vi "test.vi"() -> ()   [LabVIEW 2020]
panel:
  out "Batch Length":i32
  out "Actual Bitrate kHz 2":i32=1000
  in  "SDI":u64[](array[numeric]) format="%.0x"
  out "dup Cheetah Handle":i32
  out "Total Shifted Out":i32
  out "Actual Bitrate kHz":i32=1000
  out "error out":errorcluster
  in  "Rds per Sec":dbl=2000.0 max=2000000000.0
  out "SDO":u64[](array[numeric]) format="%x"
  in  "SCLK (kHz)":i32=2000 min=0
  out "Cheetah Handle":i32
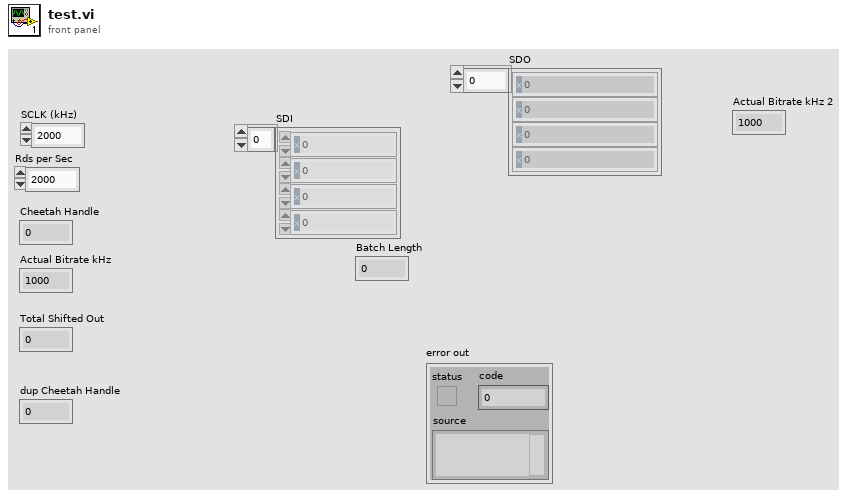
[diagram p1: front panel]
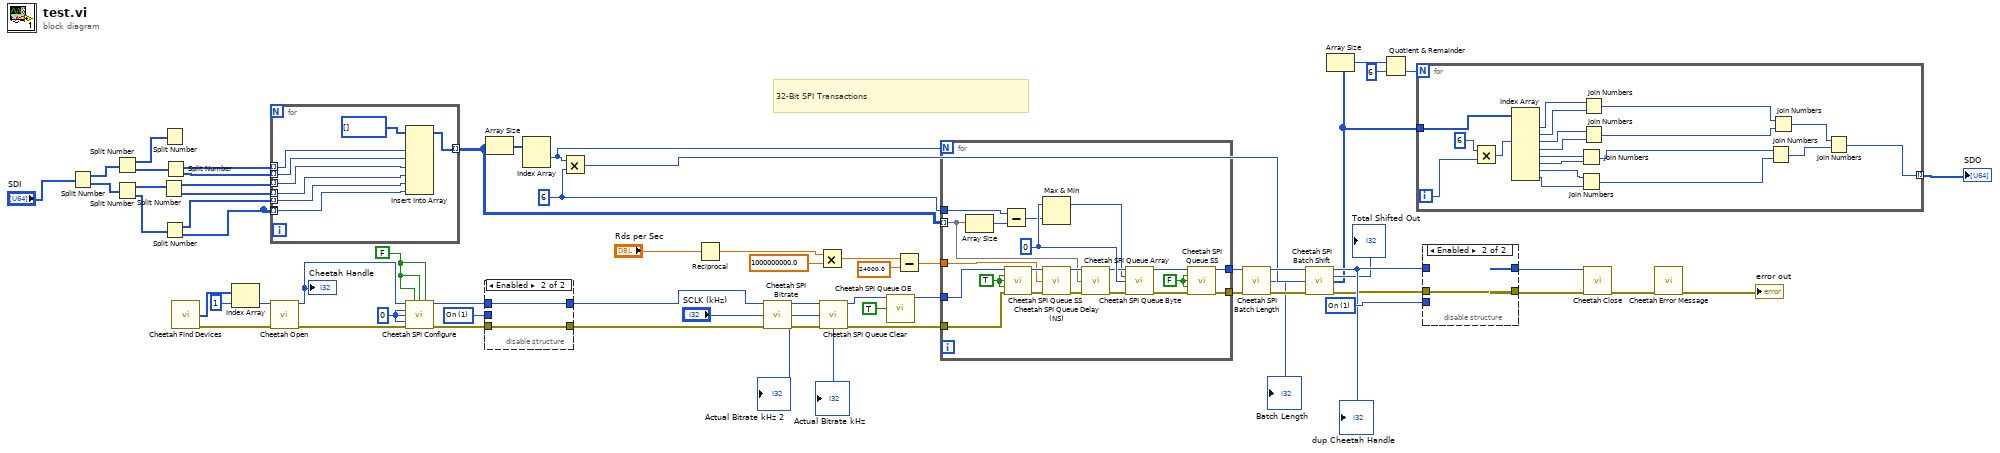
[diagram p0: block diagram]
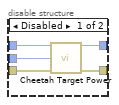
[diagram p2: hidden frame]
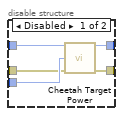
[diagram p3: hidden frame]
diagram:
  w18 = 6 ("y")
  w43 = u16 1 items=["Off", "On", "Query"] ("Requested Configuration (2: Query)")
  w44 = u16 1 items=["Off", "On", "Query"] ("Requested Configuration (2: Query)")
  w59 = FALSE
  w61 = 0
  # "32-Bit SPI Transactions"
  n1 = Split Number(x="SDI") -> (hi(x)=w29:u32[], lo(x)=w28:u32[])
  n2 = Split Number(x=w29) -> (hi(x)=w5:u16[], lo(x)=w4:u16[])
  n3 = Split Number(x=w28) -> (hi(x)=w8:u16[], lo(x)=w7:u16[])
  n4 = Split Number(x=w8) -> (hi(x)=w12:u8[], lo(x)=w11:u8[])
  n5 = Split Number(x=w5) -> ()  [unwired: 2 out]
  n6 = Split Number(x=w7) -> (hi(x)=w10:u8[], lo(x)=w9:u8[])
  n7 = Split Number(x=w4) -> (hi(x)=w3:u8[], lo(x)=w2:u8[])
  n8 = call <instrlib>:"Cheetah Find Devices.vi"() -> ("Ports"=w62:u16[], "error out"=w58:errorcluster)  [unwired: 13 in, 1 out]
  n9 = Index Array(array=w62, index=1) -> (element=w50:u16)
  n10 = for {
    tunnel: w12 -> [w67] mode=indexing
    tunnel: [w71] -> w27 mode=indexing
    tunnel: w10 -> [w65] mode=indexing
    tunnel: w9 -> [w64] mode=indexing
    tunnel: w9 -> [_] mode=indexing
    tunnel: w11 -> [w66] mode=indexing
    tunnel: w3 -> [w69] mode=indexing
    tunnel: w2 -> [w68] mode=indexing
    n11 = Insert Into Array(array=u8[] [], new element #1=w69, new element #2=w68, new element #3=w67, new element #4=w66, new element #5=w65, new element #6=w64) -> (w71:u8[])  [unwired: 1 in]
  }
  n12 = call <instrlib>:"Cheetah Open.vi"("Port Number (0)"=w50, "error in (no error)"=w58) -> ("Cheetah Handle"=w55:i32, "error out"=w57:errorcluster)  [unwired: 12 in]
  "Cheetah Handle" <- w55
  n13 = call <instrlib>:"Cheetah SPI Configure.vi"("Cheetah Handle"=w55, "SS0 Active High? (False)"=w59, "SS1 Active High? (False)"=w59, "SS2 Active High? (False)"=w59, "Polarity (0: Rising/Falling)"=w61, "Phase (0: Sample/Setup)"=w61, "Bitorder (0: MSB)"=w61, "error in (no error)"=w57) -> ("dup Cheetah Handle"=w54:i32, "error out"=w56:errorcluster)  [unwired: 6 in]
  n14 = disable-structure shown="Enabled" {
    disable-tunnel: w56 -> [w76 w77]
    disable-tunnel: w54 -> [w75 w78]
    disable-tunnel: [w74 w77] -> w53
    disable-tunnel: [w73 w78] -> w51
    disable-tunnel: w43 -> [w72 _]
    frame Disabled {
      n15 = call <instrlib>:"Cheetah Target Power.vi"("Cheetah Handle"=w75, "Requested Configuration (2: Query)"=w72, "error in (no error)"=w76) -> ("dup Cheetah Handle"=w73:i32, "error out"=w74:errorcluster)  [unwired: 10 in, 1 out]
    }
    frame Enabled {
    }
  }
  n16 = Array Size(array=w27) -> (size(s)=w42:i32[])
  n17 = Index Array(array=w42) -> (element #1=w14:i32)  [unwired: 2 in, 1 out]
  n18 = Multiply(x=w14, y=w18) -> (x*y=w13:i32)
  n19 = Reciprocal(x="Rds per Sec") -> (1/x=w20:dbl)
  n20 = call <instrlib>:"Cheetah SPI Bitrate.vi"("Cheetah Handle"=w51, "Requested Bitrate kHz (1000)"="SCLK (kHz)", "error in (no error)"=w53) -> ("dup Cheetah Handle"=w49:i32, "Actual Bitrate kHz"=→"Actual Bitrate kHz" →"Actual Bitrate kHz 2":i32, "error out"=w48:errorcluster)  [unwired: 10 in]
  n21 = Multiply(x=w20, y=1000000000.0) -> (x*y=w23:dbl)
  n22 = call <instrlib>:"Cheetah SPI Queue Clear.vi"("Cheetah Handle"=w49, "error in (no error)"=w48) -> ("dup Cheetah Handle"=w41:i32, "error out"=w60:errorcluster)  [unwired: 12 in]
  n23 = call <instrlib>:"Cheetah SPI Queue OE.vi"("Cheetah Handle"=w41, "Output Enable (on)"=TRUE) -> ("dup Cheetah Handle"=w40:i32)  [unwired: 12 in, 1 out]
  n24 = Subtract(x=w23, y=24000.0) -> (x-y=w21:dbl)
  n25 = for {
    N: w14 -> [_]
    tunnel: w60 -> [w85]
    tunnel: w40 -> [w86]
    tunnel: w27 -> [w87] mode=indexing
    tunnel: [w84] -> w38
    tunnel: [w83] -> w37
    tunnel: w21 -> [w80]
    tunnel: w18 -> [w81]
    w91 = FALSE
    w94 = 0
    w82 = TRUE
    n26 = Array Size(array=w87) -> (size(s)=w88:i32)
    n27 = Subtract(x=w81, y=w88) -> (x-y=w92:i32)
    n28 = call <instrlib>:"Cheetah SPI Queue SS.vi"("Cheetah Handle"=w86, "SS0 Assert? (True)"=w82, "SS1 Assert? (True)"=w82, "SS2 Assert? (True)"=w82, "error in (no error)"=w85) -> ("dup Cheetah Handle"=w99:i32, "error out"=w98:errorcluster)  [unwired: 9 in]
    n29 = Max & Min(x=w94, y=w92) -> (max(x,y)=w79:i32)  [unwired: 1 out]
    n30 = call <instrlib>:"Cheetah SPI Queue Delay (NS).vi"("Cheetah Handle"=w99, "Delay NS (1000)"=w80, "error in (no error)"=w98) -> ("dup Cheetah Handle"=w97:i32, "error out"=w96:errorcluster)  [unwired: 10 in, 1 out]
    n31 = call <instrlib>:"Cheetah SPI Queue Array.vi"("Cheetah Handle"=w97, "Data Out (none)"=w87, "error in (no error)"=w96) -> ("dup Cheetah Handle"=w93:i32, "error out"=w95:errorcluster)  [unwired: 11 in]
    n32 = call <instrlib>:"Cheetah SPI Queue Byte.vi"("Cheetah Handle"=w93, "Byte Count (1)"=w79, "Byte Value (0x00)"=w94, "error in (no error)"=w95) -> ("dup Cheetah Handle"=w90:i32, "error out"=w89:errorcluster)  [unwired: 10 in]
    n33 = call <instrlib>:"Cheetah SPI Queue SS.vi"("Cheetah Handle"=w90, "SS0 Assert? (True)"=w91, "SS1 Assert? (True)"=w91, "SS2 Assert? (True)"=w91, "error in (no error)"=w89) -> ("dup Cheetah Handle"=w83:i32, "error out"=w84:errorcluster)  [unwired: 9 in]
  }
  n34 = call <instrlib>:"Cheetah SPI Batch Length.vi"("Cheetah Handle"=w37, "error in (no error)"=w38) -> ("dup Cheetah Handle"=w36:i32, "Batch Length"=→"Batch Length":i32, "error out"=w35:errorcluster)  [unwired: 11 in]
  n35 = call <instrlib>:"Cheetah SPI Batch Shift.vi"("Cheetah Handle"=w36, "Max Bytes to Retrieve (256)"=w13, "error in (no error)"=w35) -> ("dup Cheetah Handle"=w34:i32, "Total Shifted Out"=→"Total Shifted Out":i32, "Data In"=w15:u8[], "error out"=w26:errorcluster)  [unwired: 9 in]
  "dup Cheetah Handle" <- w34
  n36 = Array Size(array=w15) -> (size(s)=w33:i32)
  n37 = Quotient & Remainder(x=w33, y=6) -> (floor(x/y)=w31:i32)  [unwired: 1 out]
  n38 = for {
    N: w31 -> [_]
    tunnel: w15 -> [w117]
    tunnel: [w114] -> w30 mode=indexing
    i -> [w113]
    n39 = Multiply(x=6, y=w113) -> (x*y=w115:i32)
    n40 = Index Array(array=w117, index #3=w115) -> (element #1=w103:u8, element #2=w102:u8, element #3=w101:u8, element #4=w100:u8, element #5=w112:u8, element #6=w111:u8, element #7=w110:u8, element #8=w109:u8)  [unwired: 7 in]
    n41 = Join Numbers(hi=w112, lo=w111) -> ((hi.lo)=w108:u16)
    n42 = Join Numbers(hi=w110, lo=w109) -> ((hi.lo)=w107:u16)
    n43 = Join Numbers(hi=w103, lo=w102) -> ((hi.lo)=w106:u16)
    n44 = Join Numbers(hi=w101, lo=w100) -> ((hi.lo)=w105:u16)
    n45 = Join Numbers(hi=w108, lo=w107) -> ((hi.lo)=w118:u32)
    n46 = Join Numbers(hi=w106, lo=w105) -> ((hi.lo)=w104:u32)
    n47 = Join Numbers(hi=w104, lo=w118) -> ((hi.lo)=w114:u64)
  }
  "SDO" <- w30
  n48 = disable-structure shown="Enabled" {
    disable-tunnel: [w123 _] -> w47
    disable-tunnel: [w122 w124] -> w46
    disable-tunnel: w44 -> [w121 _]
    disable-tunnel: w34 -> [w120 _]
    disable-tunnel: w26 -> [w119 w124]
    frame Disabled {
      n49 = call <instrlib>:"Cheetah Target Power.vi"("Cheetah Handle"=w120, "Requested Configuration (2: Query)"=w121, "error in (no error)"=w119) -> ("dup Cheetah Handle"=w123:i32, "error out"=w122:errorcluster)  [unwired: 10 in, 1 out]
    }
    frame Enabled {
    }
  }
  n50 = call <instrlib>:"Cheetah Close.vi"("Cheetah Handle"=w47, "error in (no error)"=w46) -> ("error out"=w45:errorcluster)  [unwired: 12 in, 1 out]
  n51 = call <instrlib>:"Cheetah Error Message.vi"("error in (no error)"=w45) -> ("error out"=→"error out":errorcluster)  [unwired: 10 in, 4 out]
